vi "20211008_exercise code.vi"() -> ()   [LabVIEW 2019]
uses:
  <vilib>/Analysis/Matrix/Datatypes/RealMatrix.ctl
  <vilib>/Analysis/baseanly.llb/Real Outer Product.vi
  <vilib>/Analysis/NI_AALBase.lvlib
  <vilib>/Analysis/Matrix/NI_Matrix.lvlib
panel:
  out "Matrix":i32[][](array[numeric])=[[1, 2, 3, 4, 5, 6, 7, 8, 9], [1, 2, 3, 4, 5, 6, 7, 8, 9], [1, 2, 3, 4, 5, 6, 7, 8, 9], [1, 2, 3, 4, 5, 6, 7, 8, 9], [1, 2, 3, 4, 5, 6, 7, 8, 9], [1, 2, 3, 4, 5, 6, 7, 8, 9], [1, 2, 3, 4, 5, 6, 7, 8, 9], [1, 2, 3, 4, 5, 6, 7, 8, 9], [1, 2, 3, 4, 5, 6, 7, 8, 9], [1, 2, 3, 4, 5, 6, 7, 8, 9], [1, 2, 3, 4, 5, 6, 7, 8, 9], [1, 2, 3, 4, 5, 6, 7, 8, 9], [1, 2, 3, 4, 5, 6, 7, 8, 9], [1, 2, 3, 4, 5, 6, 7, 8, 9], [1, 2, 3, 4, 5, 6, 7, 8, 9], [1, 2, 3, 4, 5, 6, 7, 8, 9]]
  out "Vector":i32[](array[numeric])=[1, 2, 3, 4, 5, 6, 7, 8, 9, 0, 0, 0, 0, 0, 0, 0]
  out "Array 2":i32[](array[numeric])=[0, 3, 6, 9]
  out "Array":i32[](array[numeric])=[1, 2, 3, 4, 5, 6, 7, 8, 9, 2, 4, 6, 8, 10, 12, 14, 16, 18, 3, 6, 9, 12, 15, 18, 21, 24, 27, 4, 8, 12, 16, 20, 24, 28, 32, 36, 5, 10, 15, 20, 25, 30, 35, 40, 45, 6, 12, 18, 24, 30, 36, 42, 48, 54, 7, 14, 21, 28, 35, 42, 49, 56, 63, 8, 16, 24, 32, 40, 48, 56, 64, 72, 9, 18, 27, 36, 45, 54, 63, 72, 81]
  out "matrix":i32[][](array[numeric])=[[1, 2, 3, 4, 5, 6, 7, 8, 9], [2, 4, 6, 8, 10, 12, 14, 16, 18], [3, 6, 9, 12, 15, 18, 21, 24, 27], [4, 8, 12, 16, 20, 24, 28, 32, 36], [5, 10, 15, 20, 25, 30, 35, 40, 45], [6, 12, 18, 24, 30, 36, 42, 48, 54], [7, 14, 21, 28, 35, 42, 49, 56, 63], [8, 16, 24, 32, 40, 48, 56, 64, 72], [9, 18, 27, 36, 45, 54, 63, 72, 81]]
  out "Outer Product":T1=[[1.0, 2.0, 3.0, 4.0, 5.0, 6.0, 7.0, 8.0, 9.0], [2.0, 4.0, 6.0, 8.0, 10.0, 12.0, 14.0, 16.0, 18.0], [3.0, 6.0, 9.0, 12.0, 15.0, 18.0, 21.0, 24.0, 27.0], [4.0, 8.0, 12.0, 16.0, 20.0, 24.0, 28.0, 32.0, 36.0], [5.0, 10.0, 15.0, 20.0, 25.0, 30.0, 35.0, 40.0, 45.0], [6.0, 12.0, 18.0, 24.0, 30.0, 36.0, 42.0, 48.0, 54.0], [7.0, 14.0, 21.0, 28.0, 35.0, 42.0, 49.0, 56.0, 63.0], [8.0, 16.0, 24.0, 32.0, 40.0, 48.0, 56.0, 64.0, 72.0], [9.0, 18.0, 27.0, 36.0, 45.0, 54.0, 63.0, 72.0, 81.0]]
  out "matrix":i32[][](array[numeric])=[[1, 2, 3, 4, 5, 6, 7, 8, 9], [2, 4, 6, 8, 10, 12, 14, 16, 18], [3, 6, 9, 12, 15, 18, 21, 24, 27], [4, 8, 12, 16, 20, 24, 28, 32, 36], [5, 10, 15, 20, 25, 30, 35, 40, 45], [6, 12, 18, 24, 30, 36, 42, 48, 54], [7, 14, 21, 28, 35, 42, 49, 56, 63], [8, 16, 24, 32, 40, 48, 56, 64, 72], [9, 18, 27, 36, 45, 54, 63, 72, 81]]
  out "vector":i32[](array[numeric])=[1, 2, 3, 4, 5, 6, 7, 8, 9]
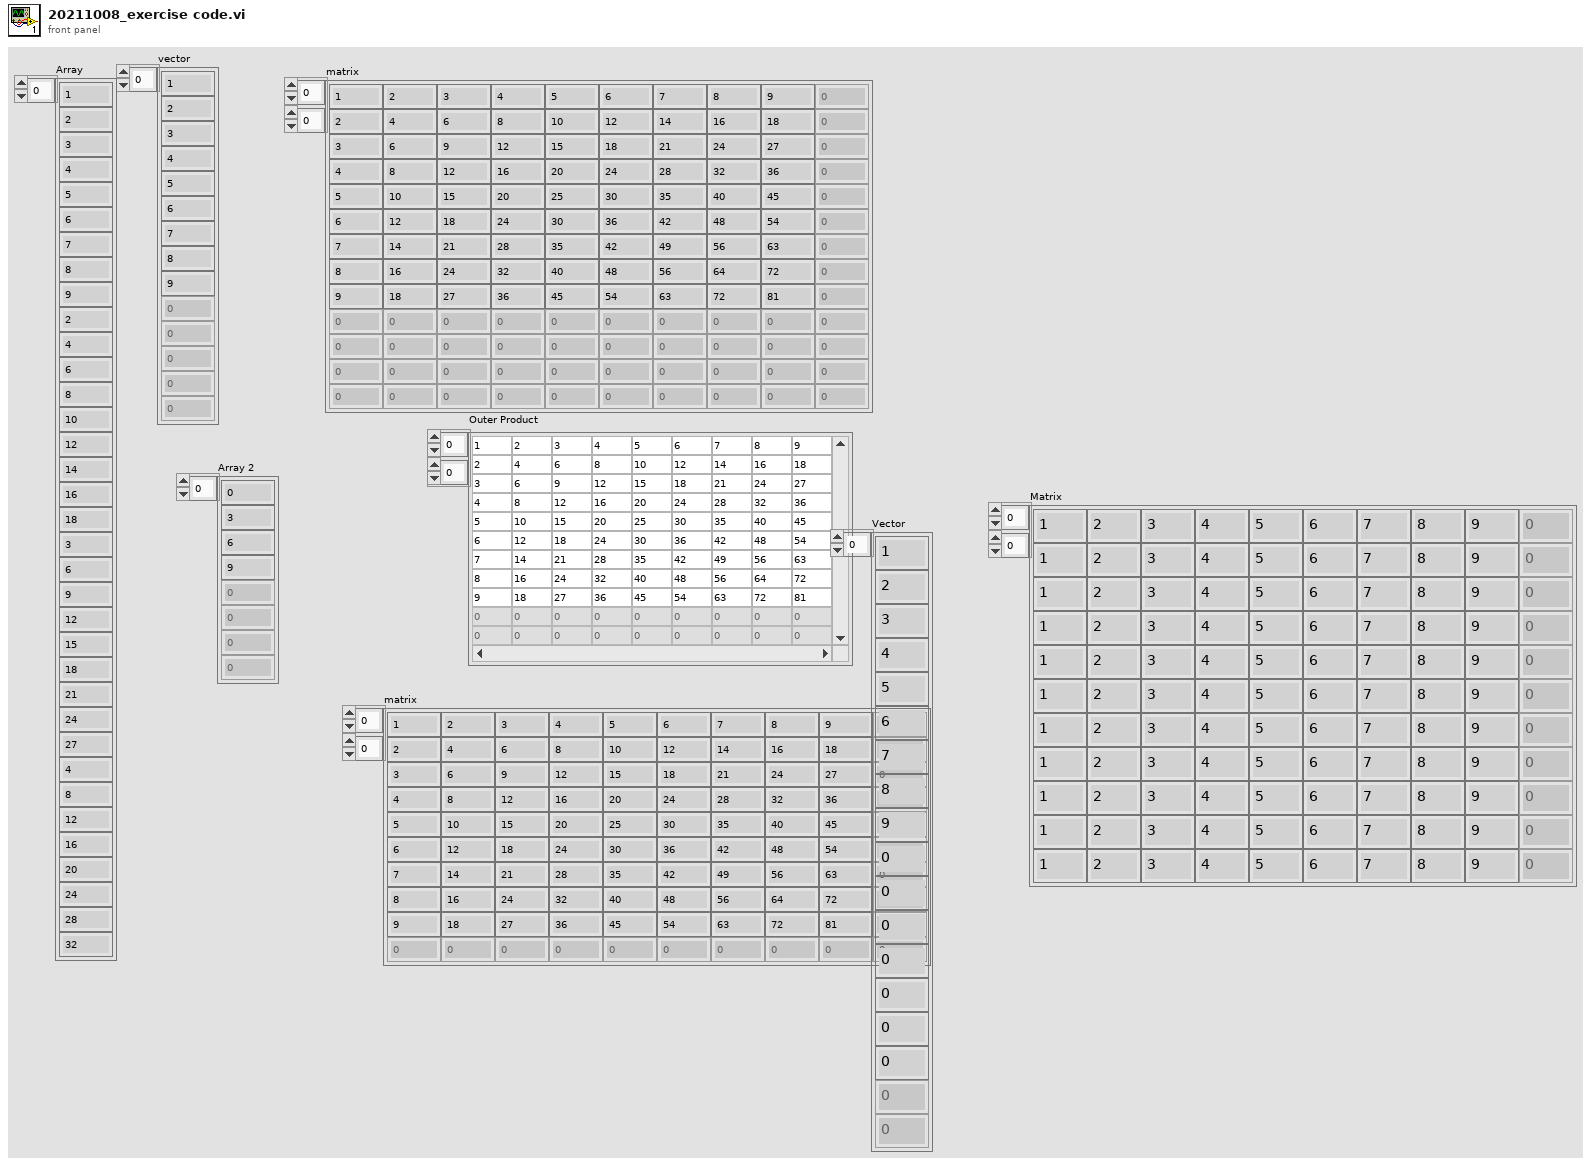
[diagram p1: front panel]
types:
  T1 = typedef "NI_Matrix.lvlib/RealMatrix.ctl" = dbl[][]
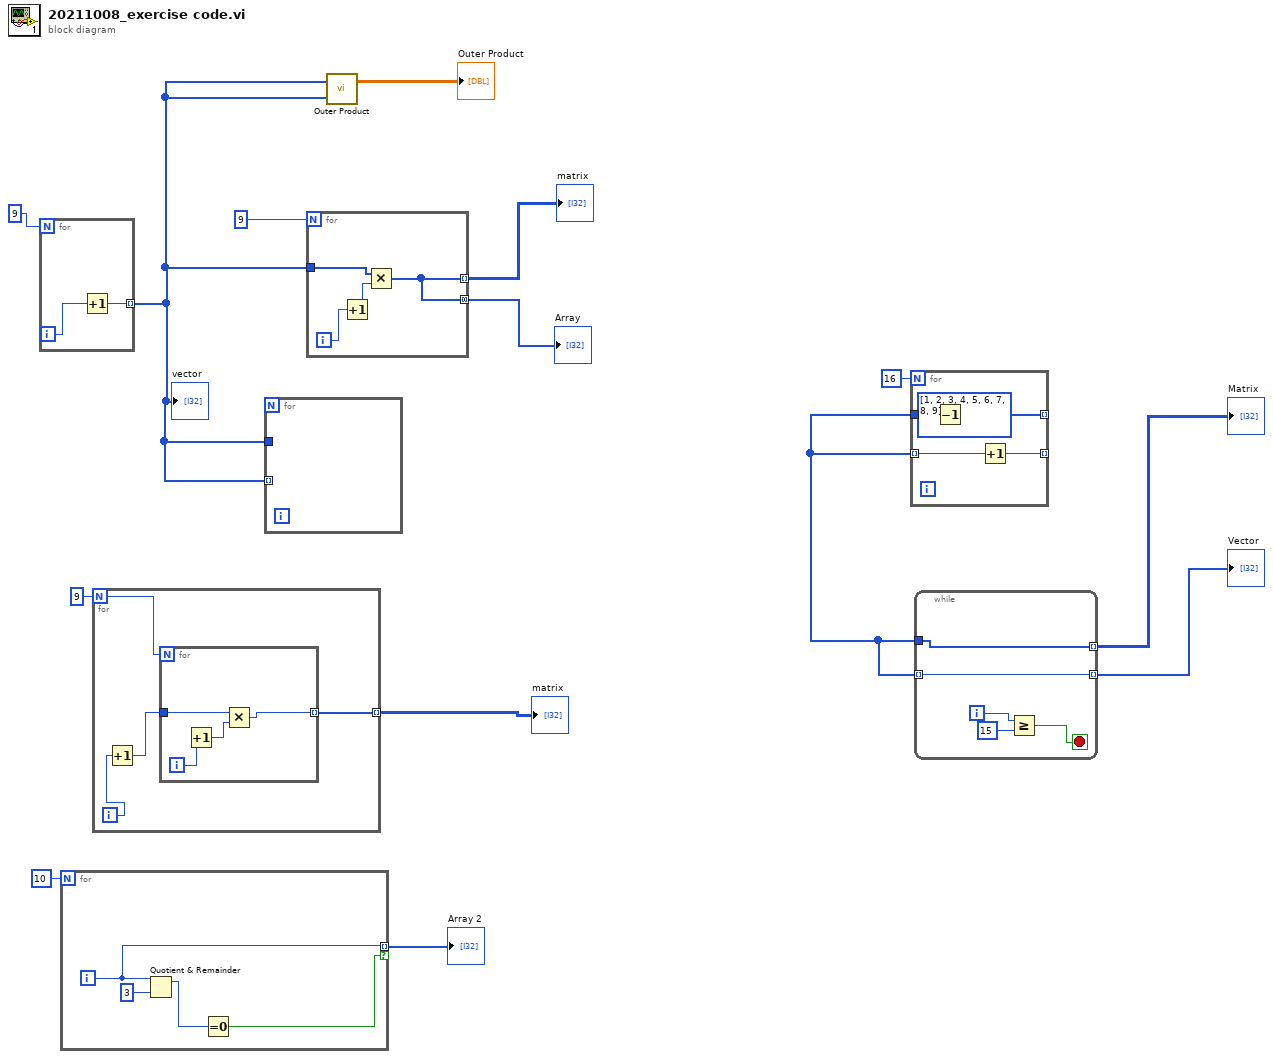
[diagram p0: block diagram]
diagram:
  w3 = i32[] [1, 2, 3, 4, 5, 6, 7, 8, 9] ("vector")
  n1 = for {
    N: 9 -> [_]
    tunnel: [w15] -> w5 mode=indexing
    i -> [w16]
    n2 = Increment(x=w16) -> (x+1=w15:i32)
  }
  "vector" <- w5
  n3 = for {
    N: 10 -> [_]
    tunnel: [w18] -> w6 mode=indexing if=w17
    i -> [w18]
    n4 = Quotient & Remainder(x=w18, y=3) -> (x-y*floor(x/y)=w19:i32)  [unwired: 1 out]
    n5 = Equal To 0?(x=w19) -> (x = 0?=w17:bool)
  }
  "Array 2" <- w6
  n6 = for {
    N: 9 -> [w24]
    tunnel: [w21] -> w9 mode=indexing
    i -> [w22]
    n7 = Increment(x=w22) -> (x+1=w23:i32)
    n8 = for {
      N: w24 -> [_]
      tunnel: w23 -> [w26]
      tunnel: [w25] -> w21 mode=indexing
      i -> [w28]
      n9 = Increment(x=w28) -> (x+1=w27:i32)
      n10 = Multiply(x=w26, y=w27) -> (x*y=w25:i32)
    }
  }
  "matrix" <- w9
  n11 = for {
    tunnel: w5 -> [_]
    tunnel: w5 -> [_] mode=indexing
  }
  n12 = for {
    N: 9 -> [_]
    tunnel: w5 -> [w31]
    tunnel: [w30] -> w12 mode=indexing
    tunnel: [w30] -> w8 mode=concatenating
    i -> [w32]
    n13 = Increment(x=w32) -> (x+1=w29:i32)
    n14 = Multiply(x=w31, y=w29) -> (x*y=w30:i32[])
  }
  "matrix" <- w12
  "Array" <- w8
  n15 = call-poly <vilib>:"Outer Product.vi"("Y Vector"=w5, "X Vector"=w5) -> ("Outer Product"=→"Outer Product":T1)  [unwired: 1 out]
  n16 = for {
    N: 16 -> [_]
    tunnel: w3 -> [w36]
    tunnel: w3 -> [w35] mode=indexing
    tunnel: [w33] -> _ mode=indexing
    tunnel: [w34] -> _ mode=indexing
    n17 = Decrement(x=w36) -> (x-1=w33:i32[])
    n18 = Increment(x=w35) -> (x+1=w34:i32)
  }
  n19 = while {
    tunnel: w3 -> [w41]
    tunnel: w3 -> [w40] mode=indexing
    tunnel: [w41] -> w2 mode=indexing
    tunnel: [w40] -> w1 mode=indexing
    i -> [w39]
    stop <- w37 stop-if-true
    n20 = Greater Or Equal?(x=w39, y=15) -> (x >= y?=w37:bool)
  }
  "Vector" <- w1
  "Matrix" <- w2
